vi "Check If Discovery Service is Running.vi"(8 "error in":errorcluster) -> (0 "error out":errorcluster, 3 "discovery service running?":bool)   [LabVIEW 2020, in "MeasurementServerTests.lvlib"]
uses:
  MeasurementServerTests.lvlib
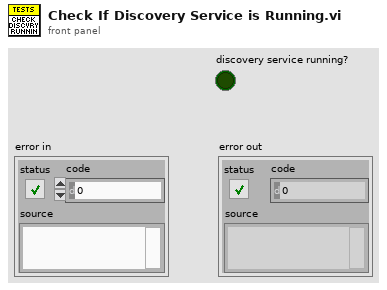
[diagram p1: front panel]
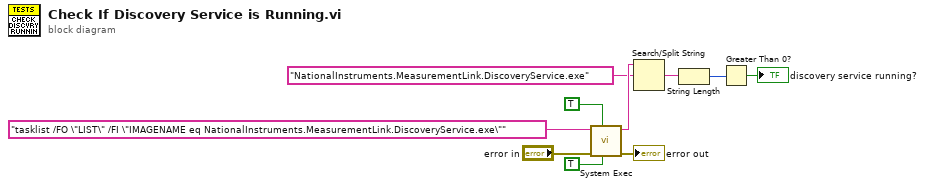
[diagram p0: block diagram]
diagram:
  n1 = call <vilib>:"System Exec.vi"("run minimized? (F)"=TRUE, "wait until completion? (T)"=TRUE, "error in (no error)"="error in", "command line"="tasklist /FO \"LIST\" /FI \"IMAGENAME eq NationalInstruments.MeasurementLink.DiscoveryService.exe\"") -> ("error out"=→"error out":errorcluster, "standard output"=w5:string)  [unwired: 4 in, 2 out]
  n2 = Search/Split String(string=w5, search string/char (-)="NationalInstruments.MeasurementLink.DiscoveryService.exe") -> (match + rest of string=w3:string)  [unwired: 1 in, 2 out]
  n3 = String Length(string=w3) -> (length=w2:i32)
  n4 = Greater Than 0?(x=w2) -> (x > 0?=→"discovery service running?":bool)
